vi "FB Switch Input Const Var Write.vi"(8 "error in":errorcluster) -> (0 "error out":errorcluster, 3 "data out":variant)   [LabVIEW 2017]
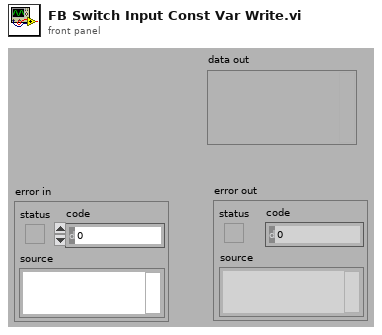
[diagram p1: front panel]
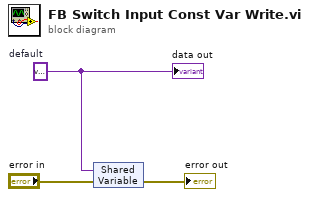
[diagram p0: block diagram]
diagram:
  w1 = variant  # default
  n1 = shared-variable(w1, error in="error in") -> (error out=→"error out":errorcluster)
  "data out" <- w1
